vi "Synchronized Acquisition.vi"() -> ()   [LabVIEW 2018, in "GettingStarted_5785_Host.lvlib"]
uses:
  GettingStarted_5785_Host.lvlib
  <vilib>/userdefined/High Color/nirio_resource_hc.ctl
  <instrlib>/FlexRIO/API/Host/v1/NI FlexRIO/API/Reference Clock Source.ctl
  <instrlib>/FlexRIO/API/Host/v1/NI FlexRIO/API/Configure Reference Clock.vi
  <instrlib>/FlexRIO/API/Host/v1/NI FlexRIO/API/Configure Immediate Start Trigger.vi
  <instrlib>/FlexRIO/API/Host/v1/NI FlexRIO/API/Configure Analog Start Trigger.vi
  <instrlib>/FlexRIO/API/Host/v1/NI FlexRIO/API/Configure Digital Edge Start Trigger.vi
  <instrlib>/FlexRIO/API/Host/v1/NI FlexRIO/API/Get Property Reference - Fpga Small.vi
  <instrlib>/FlexRIO/API/Host/v1/NI FlexRIO/API/Read Stream 1D WDT.vi
  <vilib>/FPGAPlugInAG/Dynamic/niLvFpga_Close_Dynamic.vi
  <vilib>/rvi/interface/nirviCloseFPGA/nirviCloseFPGA.xnode
  <instrlib>/FlexRIO/API/Host/v1/NI FlexRIO API v1.lvlib
  <resource>/objmgr/sessionReference.rc
  <resource>/objmgr/niflexrioapiStream.rc
panel:
  in  "reference clock source":T1 items=["Default", "Onboard", "PXI_Clk10", "External", "None", "Baseboard Reference"]
  in  "stop":bool
  out "error out":errorcluster
  out "Waveform Graph":waveform(dbl)[](graph)
  in  "acquire pretrigger \nsamples?":bool
  in  "min. TClk period":dbl=1e-06 format="%#_6p"
  in  "trigger master index":i32
  in  "Tab Control":enum32{"Immediate", "Digital", "Analog"}(tab)
  in  "trigger source":string(combo)="PXI_Trig0"
  in  "rising edge?":bool=TRUE
  in  "trigger channel":string="AI0"
  in  "level (V)":dbl
  in  "hysteresis (V)":dbl
  in  "device configuration":T3(array[cluster])=[{"FlexRIO digitizer"="RIO0", "channels"="AI0", "samples"=65536, "bitfile path"=path ""}, {"FlexRIO digitizer"="RIO1", "channels"="AI0", "samples"=65536, "bitfile path"=path ""}]
  # "Overview: Configure multiple FlexRIO targets for a synchronized acquisition using the FlexRIO Host API and NI-TClk API.\nRequirements: FlexRIO, NI-TClk\nInstructions: \n 1. Fill in the device configuration array with the resource name of the FlexRIO digitizers to synchronize, as well as the number of samples and which channels to acquire on.\n 2. Specify which device should be used as the trigger master using trigger master index\n 3. Configure the trigger settings for the master device\n 4. Optionally configure the reference clock to be used\n 5. Run the VI"
  # "Trigger Master Configuration"
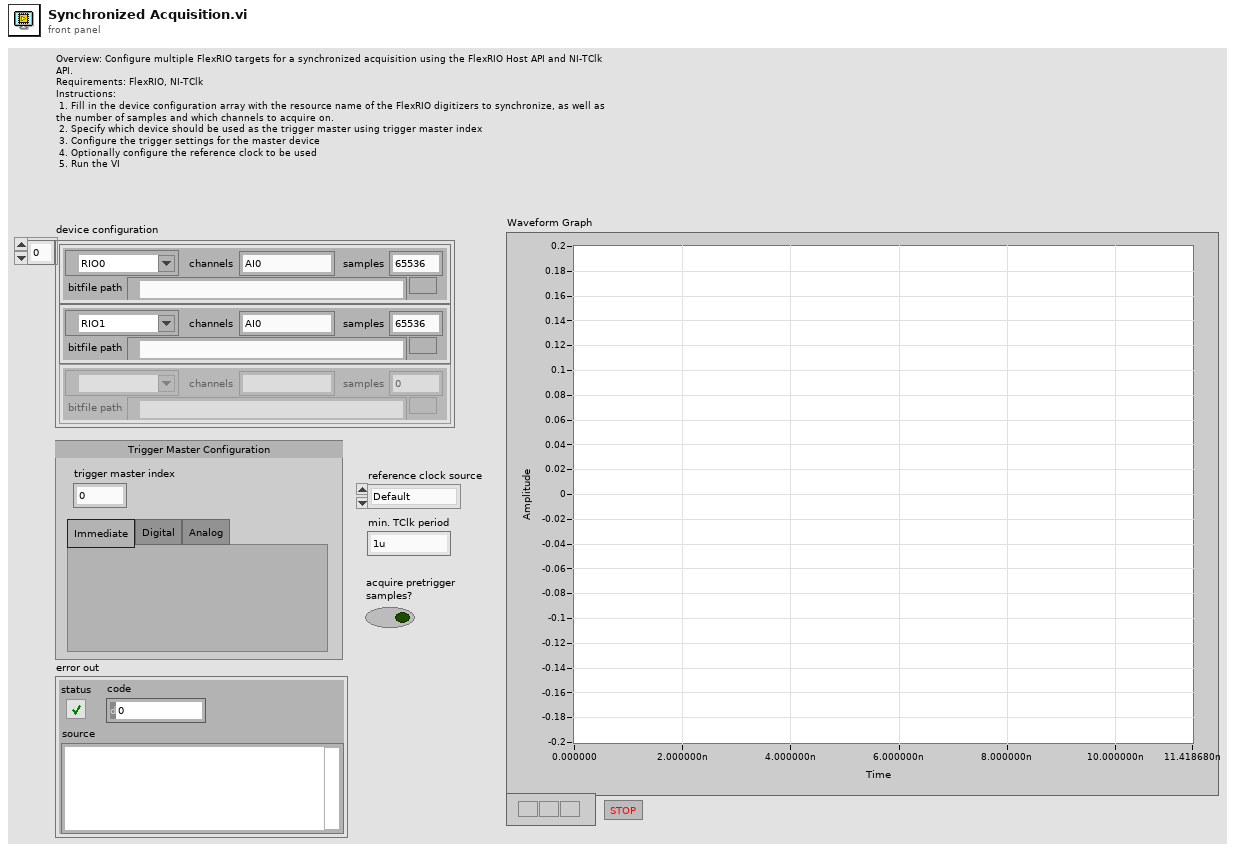
[diagram p1: front panel]
types:
  T1 = typedef "NI FlexRIO API v1.lvlib/Reference Clock Source.ctl" = i32
  T2 = typedef "nirio_resource_hc.ctl" = tag
  T3 = cluster{"FlexRIO digitizer":T2, "channels":string, "samples":u64, "bitfile path":path}[]
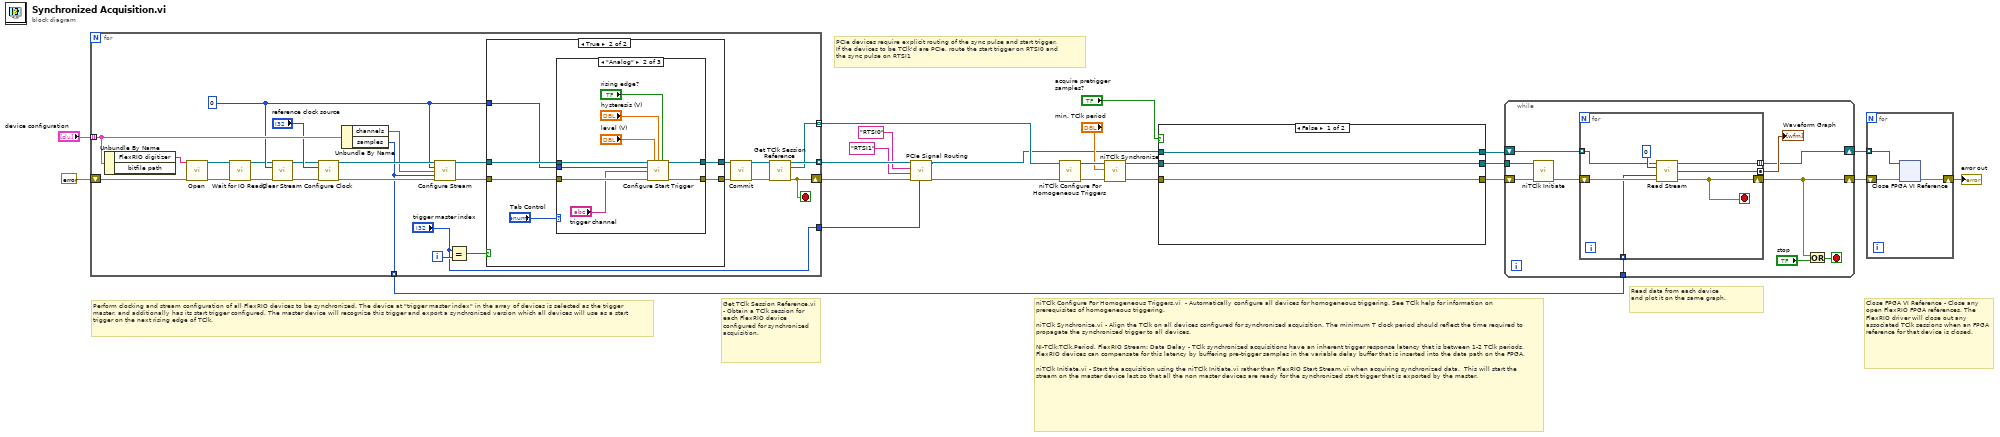
[diagram p0: block diagram]
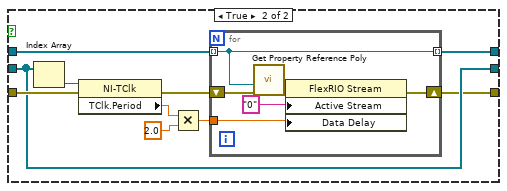
[diagram p2: hidden frame]
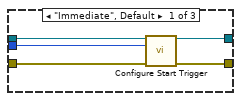
[diagram p4: hidden frame]
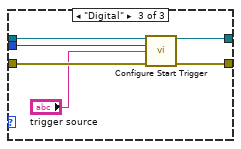
[diagram p5: hidden frame]
diagram:
  # "PCIe devices require explicit routing of the sync pulse and start trigger.\nIf the devices to be TClk'd are PCIe, route the start trigger on RTSI0 and\nthe sync pulse on RTSI1"
  # "Get TClk Session Reference.vi  - Obtain a TClk session for each FlexRIO device configured for synchronized acquisition."
  # "Perform clocking and stream configuration of all FlexRIO devices to be synchronized. The device at \"trigger master index\" in the array of devices is selected as the trigger master, and additionally has its start trigger configured. The master device will recognize this trigger and export a synchronized version which all devices will use as a start trigger on the next rising edge of TClk."
  # "niTClk Configure For Homogeneous Triggers.vi  - Automatically configure all devices for homogeneous triggering. See TClk help for information on prerequisites of homogeneous triggering. \n\nniTClk Synchronize.vi - Align the TClk on all devices configured for synchronized acquisition. The minimum T clock period should reflect the time required to propagate the synchronized trigger to all devices. \n\nNI-TClk:TClk.Period, FlexRIO Stream: Data Delay - TClk synchronized acquisitions have an inherent trigger response latency that is between 1-2 TClk periods. FlexRIO devices can compensate for this latency by buffering pre-trigger samples in the variable delay buffer that is inserted into the data path on the FPGA. \n\nniTClk Initiate.vi - Start the acquisition using the niTClk Initiate.vi rather than FlexRIO Start Stream.vi when acquiring synchronized data.  This will start the stream on the master device last so that all the non master devices are ready for the synchronized start trigger that is exported by the master."
  # "Read data from each device\nand plot it on the same graph."
  # "Close FPGA VI Reference - Close any open FlexRIO FPGA references. The FlexRIO driver will close out any associated TClk sessions when an FPGA reference for that device is closed."
  n1 = for {
    tunnel: "device configuration" -> [w46] mode=indexing
    tunnel: [w38] -> w6 mode=indexing
    tunnel: [w37] -> w11 mode=indexing
    shift-right: [w36] -> w7
    shift-left: errorcluster {"status"=FALSE, "code"=0, "source"=""} ("error out") -> [w32]
    tunnel: [w35] -> w14 mode=indexing
    tunnel: ["trigger master index"] -> w3
    i -> [w39]
    stop <- w36 stop-if-true
    w25 = u32 0 ("stream instance")
    n2 = Unbundle By Name(w46) -> ("FlexRIO digitizer"=w31:T2)  [unwired: 1 out]
    n3 = call <instrlib>:"Open.vi"("RIO Device"=w31, "error in"=w32) -> ("fpga interface out"=w30:refnum<k20>, "error out"=w29:errorcluster)  [unwired: 12 in]
    n4 = call <instrlib>:"Wait for IO Ready.vi"("fpga interface in"=w30, "error in"=w29) -> ("fpga interface out"=w24:refnum<k20>, "error out"=w28:errorcluster)  [unwired: 10 in, 2 out]
    n5 = call <instrlib>:"Clear Stream.vi"("fpga interface in"=w24, "stream instance"=w25, "error in"=w28) -> ("fpga interface out"=w27:refnum<k20>, "error out"=w26:errorcluster)  [unwired: 10 in, 1 out]
    n6 = call-poly <instrlib>:"Configure Clock.vi"("fpga interface in"=w27, "reference clock source"="reference clock source", "error in"=w26) -> ("fpga interface out"=w50:refnum<k20>, "error out"=w49:errorcluster)  [unwired: 11 in]
    n7 = Unbundle By Name(w46) -> ("channels"=w45:string, "samples"=w35:u64)
    n8 = call <instrlib>:"Configure Stream.vi"("fpga interface in"=w50, "stream instance"=w25, "channels enabled"=w45, "num samples"=w35, "error in"=w49) -> ("fpga interface out"=w47:refnum<k20>, "error out"=w48:errorcluster)  [unwired: 7 in, 2 out]
    n9 = Equal?(x="trigger master index", y=w39) -> (x = y?=w40:bool)
    n10 = case shown="True" w40 {
      tunnel: w48 -> [w51 w57]
      tunnel: w47 -> [w52 w56]
      tunnel: [w51 w55] -> w44
      tunnel: [w52 w54] -> w43
      tunnel: w25 -> [_ w53]
      frame False {
      }
      frame True {
        n11 = case shown="\"Analog\"" "Tab Control" {
          tunnel: w57 -> [w63 w72 w78]
          tunnel: [w62 w71 w77] -> w55
          tunnel: w56 -> [w61 w70 w76]
          tunnel: [w60 w69 w75] -> w54
          tunnel: w53 -> [w59 w68 w74]
          frame "Immediate", Default {
            n12 = call-poly <instrlib>:"Configure Start Trigger.vi"("fpga interface in"=w61, "trigger instance"=w59, "error in"=w63) -> ("fpga interface out"=w60:refnum<k20>, "error out"=w62:errorcluster)  [unwired: 10 in, 1 out]
          }
          frame "Analog" {
            n13 = call-poly <instrlib>:"Configure Start Trigger.vi"("fpga interface in"=w70, "level"="level (V)", "hysteresis"="hysteresis (V)", "rising edge?"="rising edge?", "trigger instance"=w68, "channel"="trigger channel", "error in"=w72) -> ("fpga interface out"=w69:refnum<k20>, "error out"=w71:errorcluster)  [unwired: 6 in, 1 out]
          }
          frame "Digital" {
            n14 = call-poly <instrlib>:"Configure Start Trigger.vi"("fpga interface in"=w76, "trigger instance"=w74, "trigger source"="trigger source", "error in"=w78) -> ("fpga interface out"=w75:refnum<k20>, "error out"=w77:errorcluster)  [unwired: 9 in, 1 out]
          }
        }
      }
    }
    n15 = call <instrlib>:"Commit.vi"("fpga interface in"=w43, "error in"=w44) -> ("fpga interface out"=w42:refnum<k20>, "error out"=w41:errorcluster)  [unwired: 12 in]
    n16 = call <instrlib>:"Get TClk Session Reference.vi"("fpga interface in"=w42, "error in"=w41) -> ("fpga interface out"=w38:refnum<k20>, "tclk session reference"=w37:refnum<k20>, "error out"=w36:errorcluster)  [unwired: 11 in]
  }
  n17 = call "PCIe Signal Routing.vi"("trigger master index"=w3, "error in"=w7, "sync pulse rtsi line"="RTSI1", "start trigger rtsi line"="RTSI0", "fpga interfaces in"=w6) -> ("error out"=w1:errorcluster, "fpga interfaces out"=w2:refnum<k20>[])  [unwired: 5 in]
  n18 = call <instrlib>:"niTClk Configure For Homogeneous Triggers.vi"("error in (no error)"=w1, "sessions"=w11) -> ("error out"=w22:errorcluster, "sessions out"=w21:refnum<k20>[])  [unwired: 8 in]
  n19 = call <instrlib>:"niTClk Synchronize.vi"("error in (no error)"=w22, "minimum T clock period"="min. TClk period", "sessions"=w21) -> ("error out"=w20:errorcluster, "sessions out"=w19:refnum<k20>[])  [unwired: 7 in]
  n20 = case shown="False" "acquire pretrigger \nsamples?" {
    tunnel: w2 -> [w81 w90]
    tunnel: [w81 w89] -> w9
    tunnel: w20 -> [w79 w88]
    tunnel: w19 -> [w80 w84]
    tunnel: [w80 w84] -> w10
    tunnel: [w79 w83] -> w18
    frame False {
    }
    frame True {
      n21 = Index Array(array=w84) -> (element=w91:refnum<k20>)  [unwired: 1 in]
      n22 = property class="NI-TClk"(reference=w91, error in=w88) -> (error out=w82:errorcluster, "TClk.Period"=w86:dbl)  [unwired: 1 out]
      n23 = Multiply(x=w86, y=2.0) -> (x*y=w85:dbl)
      n24 = for {
        tunnel: w90 -> [w92] mode=indexing
        tunnel: [w92] -> w89 mode=indexing
        tunnel: w85 -> [w96]
        shift-right: [w95] -> w83
        shift-left: w82 -> [w94]
        n25 = call-poly <instrlib>:"Get Property Reference Poly.vi"("error in (no error)"=w94, "fpga interface in"=w92) -> ("error out"=w93:errorcluster, "property reference"=w98:refnum<k20>)  [unwired: 4 in, 1 out]
        n26 = property class="FlexRIO Stream"(reference=w98, error in=w93, "Active Stream"="0", "Data Delay"=w96) -> (error out=w95:errorcluster)  [unwired: 1 out]
      }
    }
  }
  n27 = while {
    tunnel: w10 -> [w108]
    tunnel: w14 -> [w104]
    shift-right: [w99] -> w13
    shift-left: w18 -> [w107]
    shift-right: [w102] -> w8
    shift-left: w9 -> [w106]
    stop <- w101 stop-if-true
    n28 = call <instrlib>:"niTClk Initiate.vi"("error in (no error)"=w107, "sessions"=w108) -> ("error out"=w105:errorcluster)  [unwired: 8 in, 1 out]
    n29 = for {
      tunnel: w106 -> [w113] mode=indexing
      shift-right: [w109] -> w99
      shift-left: w105 -> [w114]
      tunnel: w104 -> [w112] mode=indexing
      tunnel: [w111] -> w102 mode=indexing
      tunnel: [w110] -> w103 mode=concatenating
      stop <- w109 stop-if-true
      n30 = call-poly <instrlib>:"Read Stream.vi"("fpga interface in"=w113, "stream instance"=u32 0 ("stream number"), "samples"=w112, "error in"=w114) -> ("fpga interface out"=w111:refnum<k20>, "read data"=w110:waveform(dbl)[], "error out"=w109:errorcluster)  [unwired: 7 in, 2 out]
    }
    "Waveform Graph" <- w103
    n31 = Or(x=w99, y="stop") -> (x .or. y?=w101:bool)
  }
  n32 = for {
    tunnel: w8 -> [w117] mode=indexing
    shift-right: [w116] -> w12
    shift-left: w13 -> [w118]
    n33 = xnode "Close FPGA VI Reference"("FPGA VI Reference In"=w117, "error in"=w118) -> ("error out"=w116:errorcluster)
  }
  "error out" <- w12
